vi "Maximum Power Allowed.vi"() -> ()   [LabVIEW 2014]
panel:
  in  "Maximum Power Allowed":dbl
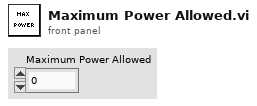
[diagram p1: front panel]
diagram:
